vi "niFPGA BW CU Order 4 (16-bit).vi"(0 "filter state in":T1, 1 "reset":bool, 5 "input data":i16, 7 "accumulator in":i32, 9 "adder in":i32, 11 "iteration":u8, 12 "in shift":i8=-1, 13 "lowpass?":bool) -> (4 "filter state out":T1, 6 "state to multiply":i32, 8 "accumulator out":i32, 10 "adder out":i32, 15 "terminate":bool)   [LabVIEW 2017]
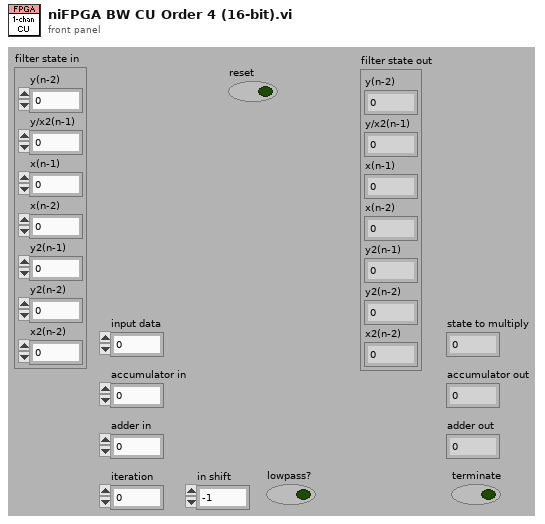
[diagram p1: front panel]
types:
  T1 = cluster{"y(n-2)":i32, "y/x2(n-1)":i32, "x(n-1)":i16, "x(n-2)":i16, "y2(n-1)":i32, "y2(n-2)":i32, "x2(n-2)":i32}
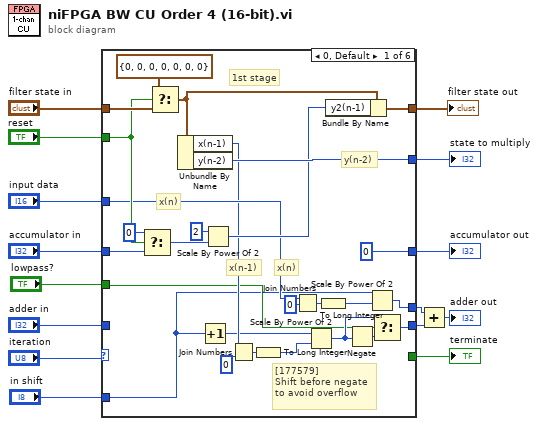
[diagram p0: block diagram]
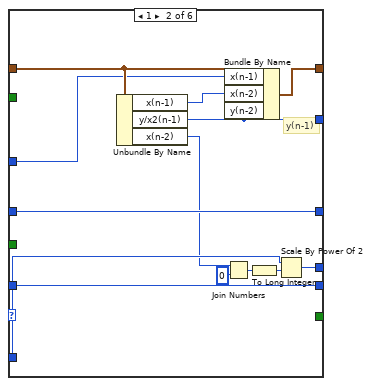
[diagram p2: hidden frame]
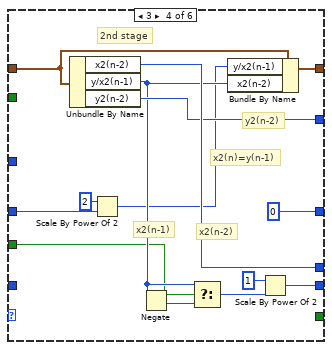
[diagram p4: hidden frame]
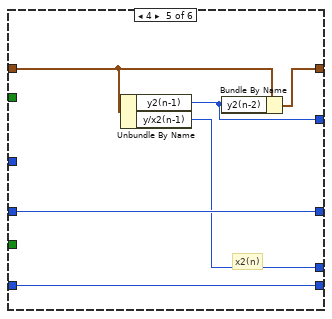
[diagram p5: hidden frame]
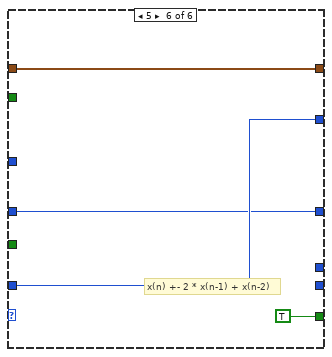
[diagram p6: hidden frame]
diagram:
  n1 = case shown="0, Default" "iteration" {
    tunnel: [w42 w52 w56 w72 w74 w79] -> w2
    tunnel: "input data" -> [w27 w51 _ _ _ _]
    tunnel: [w16 w55 _ w71 w78 _] -> w9
    tunnel: "adder in" -> [_ w55 w58 _ w78 w82]
    tunnel: [w39 w43 w58 w67 w76 w82] -> w11
    tunnel: [w26 w44 _ w69 w73 _] -> w3
    tunnel: [0 ("Numeric") w54 w57 0 ("Numeric") w77 w80] -> w10
    tunnel: [_ _ _ _ _ TRUE] -> w8
    tunnel: "reset" -> [w31 _ _ _ _ _]
    tunnel: "accumulator in" -> [w33 w54 w57 w61 w77 w80]
    tunnel: "filter state in" -> [w32 w53 w56 w62 w75 w79]
    tunnel: "in shift" -> [w19 w49 _ _ _ _]
    tunnel: "lowpass?" -> [w20 _ _ w64 _ _]
    frame 0, Default {
      # "[177579]\nShift before negate\nto avoid overflow"
      # "x(n)"
      # "1st stage"
      # "x(n)"
      # "x(n-1)"
      # "y(n-2)"
      n2 = Select(t=0, s=w31, f=w33) -> (s? t:f=w34:i32)
      n3 = Select(t=T1 {"y(n-2)"=0, "y/x2(n-1)"=0, "x(n-1)"=0, "x(n-2)"=0, "y2(n-1)"=0, "y2(n-2)"=0, "x2(n-2)"=0}, s=w31, f=w32) -> (s? t:f=w36:T1)
      n4 = Unbundle By Name(w36) -> ("x(n-1)"=w22:i16, "y(n-2)"=w39:i32)
      n5 = Increment(x=w19) -> (x+1=w18:i8)
      n6 = Scale By Power Of 2(n=2, x=w34) -> (x*2^n=w38:i32)
      n7 = Join Numbers(hi=w22, lo=i16 0) -> ((hi.lo)=w23:u32)
      n8 = To Long Integer(number=w23) -> (32bit integer=w17:i32)
      n9 = Join Numbers(hi=w27, lo=i16 0) -> ((hi.lo)=w29:u32)
      n10 = Scale By Power Of 2(n=w18, x=w17) -> (x*2^n=w21:i32)
      n11 = To Long Integer(number=w29) -> (32bit integer=w28:i32)
      n12 = Bundle By Name(cluster=w36, "y2(n-1)"=w38) -> (w42:T1)
      n13 = Negate(x=w21) -> (-x=w25:i32)
      n14 = Scale By Power Of 2(n=w19, x=w28) -> (x*2^n=w26:i32)
      n15 = Select(t=w21, s=w20, f=w25) -> (s? t:f=w16:i32)
    }
    frame 1 {
      # "y(n-1)"
      n16 = Unbundle By Name(w53) -> ("x(n-1)"=w50:i16, "y/x2(n-1)"=w43:i32, "x(n-2)"=w47:i16)
      n17 = Join Numbers(hi=w47, lo=i16 0) -> ((hi.lo)=w46:u32)
      n18 = Bundle By Name(cluster=w53, "x(n-1)"=w51, "x(n-2)"=w50, "y(n-2)"=w43) -> (w52:T1)
      n19 = To Long Integer(number=w46) -> (32bit integer=w45:i32)
      n20 = Scale By Power Of 2(n=w49, x=w45) -> (x*2^n=w44:i32)
    }
    frame 2 {
      # "x(n) +- 2 * x(n-1) + x(n-2)"
    }
    frame 3 {
      # "2nd stage"
      # "x2(n)=y(n-1)"
      # "x2(n-2)"
      # "x2(n-1)"
      # "y2(n-2)"
      n21 = Unbundle By Name(w62) -> ("x2(n-2)"=w69:i32, "y/x2(n-1)"=w65:i32, "y2(n-2)"=w67:i32)
      n22 = Scale By Power Of 2(n=2, x=w61) -> (x*2^n=w60:i32)
      n23 = Negate(x=w65) -> (-x=w66:i32)
      n24 = Select(t=w65, s=w64, f=w66) -> (s? t:f=w63:i32)
      n25 = Bundle By Name(cluster=w62, "y/x2(n-1)"=w60, "x2(n-2)"=w65) -> (w72:T1)
      n26 = Scale By Power Of 2(n=1, x=w63) -> (x*2^n=w71:i32)
    }
    frame 4 {
      # "x2(n)"
      n27 = Unbundle By Name(w75) -> ("y2(n-1)"=w76:i32, "y/x2(n-1)"=w73:i32)
      n28 = Bundle By Name(cluster=w75, "y2(n-2)"=w76) -> (w74:T1)
    }
    frame 5 {
      # "x(n) +- 2 * x(n-1) + x(n-2)"
    }
  }
  "state to multiply" <- w11
  "terminate" <- w8
  "accumulator out" <- w10
  "filter state out" <- w2
  n29 = Add(x=w3, y=w9) -> (x+y=→"adder out":i32)
